vi "Get Velocity.vi"(8 "error in (no error)":errorcluster, 11 "DC Motor Controller in":refnum<class "DC Motor Controller.lvclass">) -> (0 "error out":errorcluster, 2 "CCW Velocity (rad/s)":dbl, 3 "DC Motor Controller out":refnum<class "DC Motor Controller.lvclass">)   [LabVIEW 2019, in "DC Motor Controller.lvclass"]
doc: "Queries the counterclockwise velocity from the motor encoder."
uses:
  DC Motor Controller.lvclass
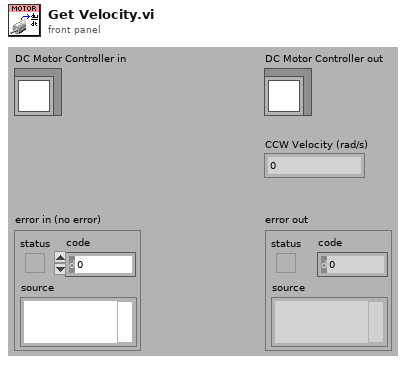
[diagram p1: front panel]
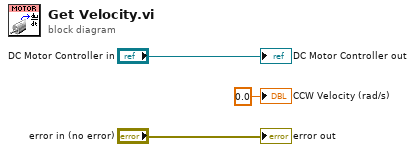
[diagram p0: block diagram]
diagram:
  "error out" <- "error in (no error)"
  "DC Motor Controller out" <- "DC Motor Controller in"
  "CCW Velocity (rad/s)" <- 0.0 ("Velocity (rad/s)")
